vi "Actor Core.vi"(8 "error in":errorcluster, 11 "Square in":refnum<class "Rigol DG822 Square.lvclass">) -> (0 "error out":errorcluster, 3 "Actor out":refnum<class "Actor.lvclass">)   [LabVIEW 2021, in "Rigol DG822 UI.lvlib" / "Rigol DG822 Square.lvlib" / "Rigol DG822 Square.lvclass"]
uses:
  Rigol DG822 Square.lvclass
  D:/LabVIEW/General/Files/lvlibp/Actors.lvlibp/Actors/Actors/Actors.lvclass
  General/Files/lvlibp/Actor Framework.lvlibp/1abvi3w/vi.lib/ActorFramework/Actor/Actor.lvclass
  Rigol DG822 UI/lib/controls.llb/FreqUnitHandler.ctl
  Rigol DG822 UI/lib/controls.llb/DataCluster.ctl
  Rigol DG822 UI/lib/controls.llb/PeriodUnitHandler.ctl
  Rigol DG822 UI/lib/controls.llb/AmplUnitHandler.ctl
  Rigol DG822 UI/lib/controls.llb/HighLUnitHandler.ctl
  Rigol DG822 UI/lib/controls.llb/OffsetUnitHandler.ctl
  Rigol DG822 UI/lib/controls.llb/LowLUnitHandler.ctl
  Rigol DG822 UI/lib/controls.llb/FreqUnit.ctl
  Rigol DG822 UI/lib/controls.llb/PeriodUnit.ctl
  Rigol DG822 UI/lib/controls.llb/AmplUnit.ctl
  Rigol DG822 UI/lib/controls.llb/HighLUnit.ctl
  Rigol DG822 UI/lib/controls.llb/OffsetUnit.ctl
  Rigol DG822 UI/lib/controls.llb/LowLUnit.ctl
  Rigol DG822 UI/lib/controls.llb/WaveformParamTags.ctl
  Rigol DG822 UI/lib/controls.llb/SquareParamDisplay.ctl
  Rigol DG822 UI/lib/controls.llb/SliderControl.ctl
  Rigol DG822 UI/lib/controls.llb/PhaseUnitHandler.ctl
  Rigol DG822 UI/lib/controls.llb/DutyUnitHandler.ctl
  Rigol DG822 UI/lib/controls.llb/StringIndicatorSelected.ctl
  Rigol DG822 UI/lib/controls.llb/RDG822ExtCall.ctl
  Rigol DG822 UI/lib/controls.llb/FT Controls Cluster.ctl
  Rigol DG822 Square.lvclass/Rigol DG822 Square.ctl
  Rigol DG822 UI/lib/controls.llb/WaveformExtCall.ctl
  Rigol DG822 UI/lib/controls.llb/AllWaveformDataCluster.ctl
  Rigol DG822 UI/lib/controls.llb/String Indicators Cluster.ctl
  <vilib>/Utility/miscctls.llb/LVPointTypeDef.ctl
  <userlib>/_MGI/Application Control/MGI VI Reference/MGI Current VI's Reference.vi
  General/Files/lvlibp/Actors.lvlibp/Actors/Actors/Actors.lvclass
panel:
  in  "Slider":T1
  in  "ParamTags":T2
  out "Data":T3={"Freq"={"Freq"=1.0, "FreqUnit"=enum."kHz", "FreqUnitPrcs"=9.0}, "Period"={"Period"=1.0, "PeriodUnit"=enum."ms", "PeriodUnitPrcs"=7.0}, "Ampl"={"Ampl"=5.0, "AmplUnit"=enum."Vpp", "AmplUnitPrcs"=4.0}, "HighL"={"HighL"=2.5, "HighLUnit"=enum."V", "HighLUnitPrcs"=4.0}, "Offset"={"Offset"=0.0, "OffsetUnit"=enum."Vdc", "OffsetUnitPrcs"=4.0}, "LowL"={"LowL"=-2.5, "LowLUnit"=enum."V", "LowLUnitPrcs"=4.0}, "Phase"={"Phase"=0.0, "PhaseUnit"=enum."°", "PhaseUnitPrcs"=3.0}, "Duty"={"Duty"=50.0, "DutyUnit"=enum."%", "DutyUnitPrcs"=3.0}, "Width"={"Width"=500.0, "WidthUnit"=enum."us", "WidthUnitPrcs"=4.0}, "RisEdge"={"RisEdge"=10.0, "RisEdgeUnit"=enum."ns", "RisEdgeUnitPrcs"=1.0}, "FallEdge"={"FallEdge"=10.0, "FallEdgeUnit"=enum."ns", "FallEdgeUnitPrcs"=1.0}} {"RisEdge"."RisEdge" format="%.1f"; "RisEdge"."RisEdgeUnitPrcs" format="%#_1g"; "FallEdge"."FallEdge" format="%.1f"; "FallEdge"."FallEdgeUnitPrcs" format="%#_1g"; "Width"."Width" format="%.4g"; "Width"."WidthUnitPrcs" format="%#_1g"; "Duty"."Duty" format="%.3g"; "Duty"."DutyUnitPrcs" format="%#_1g"; "Phase"."Phase" format="%.3g"; "Phase"."PhaseUnitPrcs" format="%#_1g"; "LowL"."LowL" format="%.4g"; "LowL"."LowLUnitPrcs" format="%#_1g"; "Offset"."Offset" format="%.4g"; "Offset"."OffsetUnitPrcs" format="%#_1g"; "HighL"."HighL" format="%.4g"; "HighL"."HighLUnitPrcs" format="%#_1g"; "Ampl"."Ampl" format="%.4g"; "Ampl"."AmplUnitPrcs" format="%#_1g"; "Period"."Period" format="%.7g"; "Period"."PeriodUnitPrcs" format="%#_1g"; "Freq"."FreqUnitPrcs" format="%#_1g"; "Freq"."Freq" format="%.9g"}
  in  "Conf Tabs":enum32{"Square", "OK"}(tab)
  in  "Slider Tab":enum32{"First", "Second"}(tab)
  in  "F/T Ctrls":T4
  out "String Indcs":T5={"Freq-Period"="1.000,000,000 kHz", "Ampl-HighL"="5.000,0 Vpp", "Offset-LowL"="0.000,0 Vdc", "Phase"="0.000 °"}
  out "F/T Ctrls 2":cluster{"Pict Ring":u16}
  out "String Indcs 2":cluster{"Duty":string}={"Duty"="50.000 %"}
  out "SquareParamDisplay":T6
  in  "Value":dbl=1.0 format="%.8g"
  in  "Unit Tabs":T7(tab)
  out "FreqUnitHandler":T8=1
  in  "FreqUnit":T9=enum."kHz"
  out "PeriodUnitHandler":T10=1
  in  "PeriodUnit":T11=enum."ms"
  in  "AmplUnit":T12=enum."Vpp"
  out "AmplUnitHandler":T13
  out "HighLUnitHandler":T14
  in  "HighLUnit":T15=enum."V"
  out "OffsetUnitHandler":T16
  in  "OffsetUnit":T17=enum."Vdc"
  out "LowLUnitHandler":T18
  in  "LowLUnit":T19=enum."V"
  out "PhaseUnitHandler":T20
  out "DutyUnitHandler":T21
  in  "OK":bool
  # "MHz - 10 \nkHz - 9\nHz - 6\nmHz - 3\nuHz - 0?"
  # "s - 10\nms - 7\nus - 4 \nns - 1?"
  # "All 4 - V - 4\n        mV - 1"
  # "no change"
  # "no change"
  # "s - 10\nms - 7\nus - 4 \nns - 1?"
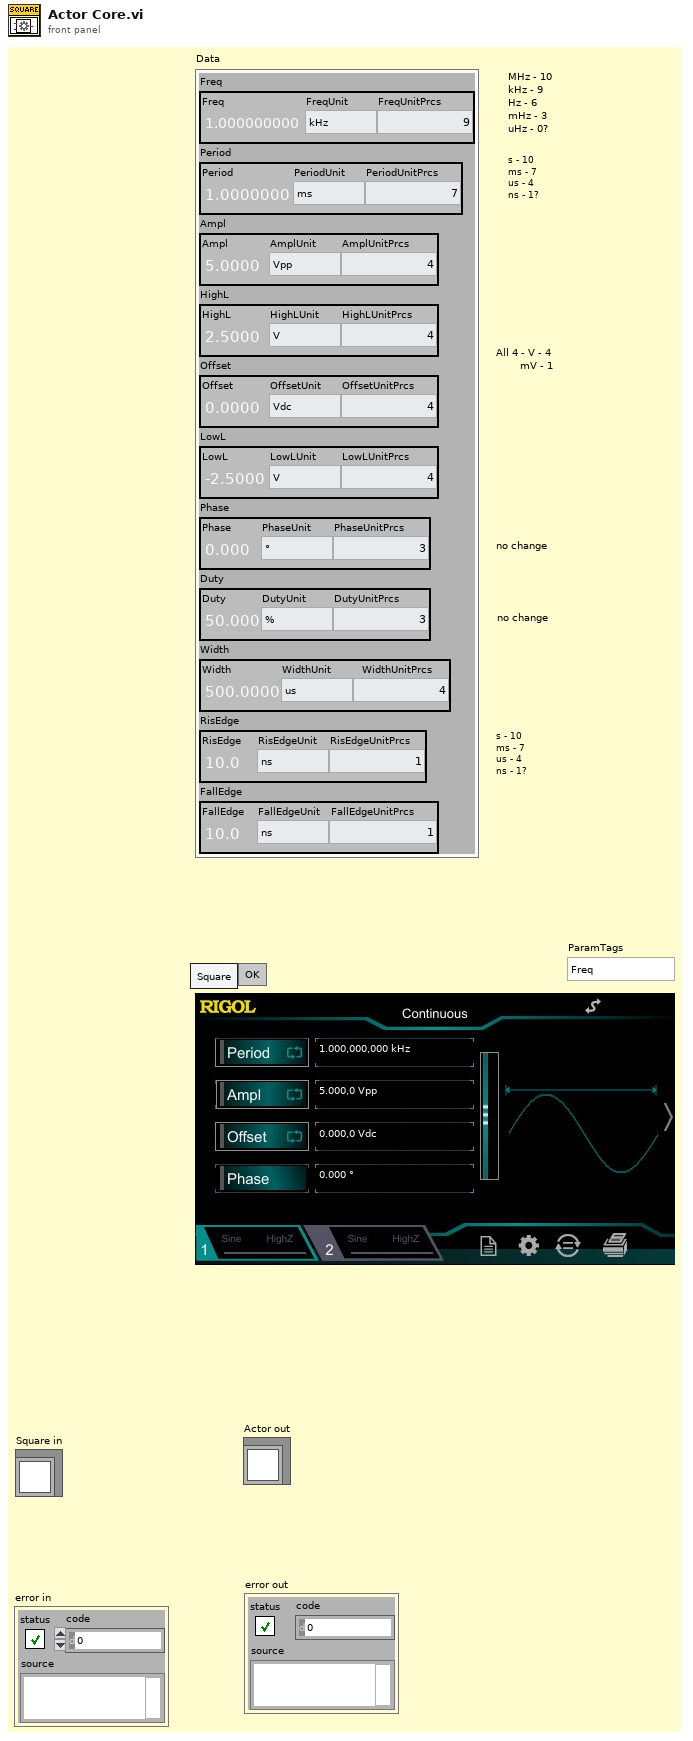
[diagram p1: front panel]
types:
  T1 = typedef "SliderControl.ctl" = bool
  T2 = typedef "WaveformParamTags.ctl" = enum16{"Freq", "Period", "Ampl", "HighL", "Offset", "LowL", "Phase", "Duty", "Width", "RisEdge", "FallEdge"}
  T3 = typedef "DataCluster.ctl" = cluster{"Freq":cluster{"Freq":dbl, "FreqUnit":enum32{"No Selection", "MHz", "kHz", "Hz", "mHz", "uHz"}, "FreqUnitPrcs":dbl}, "Period":cluster{"Period":dbl, "PeriodUnit":enum32{"No Selection", "s", "ms", "us", "ns"}, "PeriodUnitPrcs":dbl}, "Ampl":cluster{"Ampl":dbl, "AmplUnit":enum32{"No Selection", "Vpp", "mVpp"}, "AmplUnitPrcs":dbl}, "HighL":cluster{"HighL":dbl, "HighLUnit":enum32{"No Selection", "V", "mV"}, "HighLUnitPrcs":dbl}, "Offset":cluster{"Offset":dbl, "OffsetUnit":enum32{"No Selection", "Vdc", "mVdc"}, "OffsetUnitPrcs":dbl}, "LowL":cluster{"LowL":dbl, "LowLUnit":enum32{"No Selection", "V", "mV"}, "LowLUnitPrcs":dbl}, "Phase":cluster{"Phase":dbl, "PhaseUnit":enum32{"°"}, "PhaseUnitPrcs":dbl}, "Duty":cluster{"Duty":dbl, "DutyUnit":enum32{"%"}, "DutyUnitPrcs":dbl}, "Width":cluster{"Width":dbl, "WidthUnit":enum32{"No Selection", "s", "ms", "us", "ns"}, "WidthUnitPrcs":dbl}, "RisEdge":cluster{"RisEdge":dbl, "RisEdgeUnit":enum32{"No Selection", "s", "ms", "us", "ns"}, "RisEdgeUnitPrcs":dbl}, "FallEdge":cluster{"FallEdge":dbl, "FallEdgeUnit":enum32{"No Selection", "s", "ms", "us", "ns"}, "FallEdgeUnitPrcs":dbl}}
  T4 = cluster{"Freq/Period":bool, "Ampl/HighL":bool, "Offset/LowL":bool}
  T5 = cluster{"Freq-Period":string, "Ampl-HighL":string, "Offset-LowL":string, "Phase":string}
  T6 = typedef "SquareParamDisplay.ctl" = u16
  T7 = enum32{"Freq", "Period", "Ampl", "HighL", "Offset", "LowL", "Phase", "Duty"}
  T8 = typedef "FreqUnitHandler.ctl" = u16
  T9 = typedef "FreqUnit.ctl" = enum32{"No Selection", "MHz", "kHz", "Hz", "mHz", "uHz"}
  T10 = typedef "PeriodUnitHandler.ctl" = u16
  T11 = typedef "PeriodUnit.ctl" = enum32{"No Selection", "s", "ms", "us", "ns"}
  T12 = typedef "AmplUnit.ctl" = enum32{"No Selection", "Vpp", "mVpp"}
  T13 = typedef "AmplUnitHandler.ctl" = u16
  T14 = typedef "HighLUnitHandler.ctl" = u16
  T15 = typedef "HighLUnit.ctl" = enum32{"No Selection", "V", "mV"}
  T16 = typedef "OffsetUnitHandler.ctl" = u16
  T17 = typedef "OffsetUnit.ctl" = enum32{"No Selection", "Vdc", "mVdc"}
  T18 = typedef "LowLUnitHandler.ctl" = u16
  T19 = typedef "LowLUnit.ctl" = enum32{"No Selection", "V", "mV"}
  T20 = typedef "PhaseUnitHandler.ctl" = u16
  T21 = typedef "DutyUnitHandler.ctl" = u16
  T22 = cluster{"Freq-Period":string, "Freq-Period 2":string, "Freq-Period 3":string, "Freq-Period 4":string, "Freq-Period 5":string}
  T23 = typedef "LVPointTypeDef.ctl" = cluster{"Horizontal":i16, "Vertical":i16}
  T24 = typedef "StringIndicatorSelected.ctl" = enum16{"Freq-Period", "Ampl-HighL", "Offset-LowL", "Phase", "Duty-Width", "RisEdge", "FallEdge"}
  T25 = typedef "FT Controls Cluster.ctl" = cluster{"Freq/Period":bool, "Ampl/HighL":bool, "Offset/LowL":bool, "Duty/Width":bool}
  T26 = typedef "RDG822ExtCall.ctl" = enum16{"Get Data"}
  T27 = typedef "WaveformExtCall.ctl" = enum16{"Freq", "Period", "Ampl", "HighL", "Offset", "LowL", "Phase", "Duty", "Width", "RisEdge", "FallEdge", "Home", "InitData"}
  T28 = cluster{"Freq":cluster{"Freq":dbl, "FreqUnit":enum32{"No Selection", "MHz", "kHz", "Hz", "mHz", "uHz"}, "FreqUnitPrcs":dbl}, "Period":cluster{"Period":dbl, "PeriodUnit":enum32{"No Selection", "s", "ms", "us", "ns"}, "PeriodUnitPrcs":dbl}, "Duty":cluster{"Duty":dbl, "DutyUnit":enum32{"%"}, "DutyUnitPrcs":dbl}}
  T29 = cluster{"Ampl":cluster{"Ampl":dbl, "AmplUnit":enum32{"No Selection", "Vpp", "mVpp"}, "AmplUnitPrcs":dbl}, "HighL":cluster{"HighL":dbl, "HighLUnit":enum32{"No Selection", "V", "mV"}, "HighLUnitPrcs":dbl}, "Offset":cluster{"Offset":dbl, "OffsetUnit":enum32{"No Selection", "Vdc", "mVdc"}, "OffsetUnitPrcs":dbl}, "LowL":cluster{"LowL":dbl, "LowLUnit":enum32{"No Selection", "V", "mV"}, "LowLUnitPrcs":dbl}}
  T30 = cluster{"Phase":dbl, "PhaseUnit":enum32{"°"}, "PhaseUnitPrcs":dbl}
  T31 = cluster{"Duty":dbl, "DutyUnit":enum32{"%"}, "DutyUnitPrcs":dbl}
  T32 = typedef "AllWaveformDataCluster.ctl" = cluster{"Data":T3, "F/T Ctrls":T25, "String Indcs":T33}
  T33 = typedef "String Indicators Cluster.ctl" = cluster{"Freq-Period":string, "Ampl-HighL":string, "Offset-LowL":string, "Phase":string, "Duty-Width":string, "RisEdge":string, "FallEdge":string}
  T34 = enum32{"No Selection", "MHz", "kHz", "Hz", "mHz", "uHz"}
  T35 = cluster{"Value":dbl, "PeriodUnit":u32, "FreqUnitPrecision":dbl}
  T36 = cluster{"Freq":dbl, "FreqUnit":enum32{"No Selection", "MHz", "kHz", "Hz", "mHz", "uHz"}, "FreqUnitPrcs":dbl}
  T37 = cluster{"Period":dbl, "PeriodUnit":enum32{"No Selection", "s", "ms", "us", "ns"}, "PeriodUnitPrcs":dbl}
  T38 = cluster{"Ampl":dbl, "AmplUnit":enum32{"No Selection", "Vpp", "mVpp"}, "AmplUnitPrcs":dbl}
  T39 = cluster{"HighL":dbl, "HighLUnit":enum32{"No Selection", "V", "mV"}, "HighLUnitPrcs":dbl}
  T40 = cluster{"Offset":dbl, "OffsetUnit":enum32{"No Selection", "Vdc", "mVdc"}, "OffsetUnitPrcs":dbl}
  T41 = cluster{"LowL":dbl, "LowLUnit":enum32{"No Selection", "V", "mV"}, "LowLUnitPrcs":dbl}
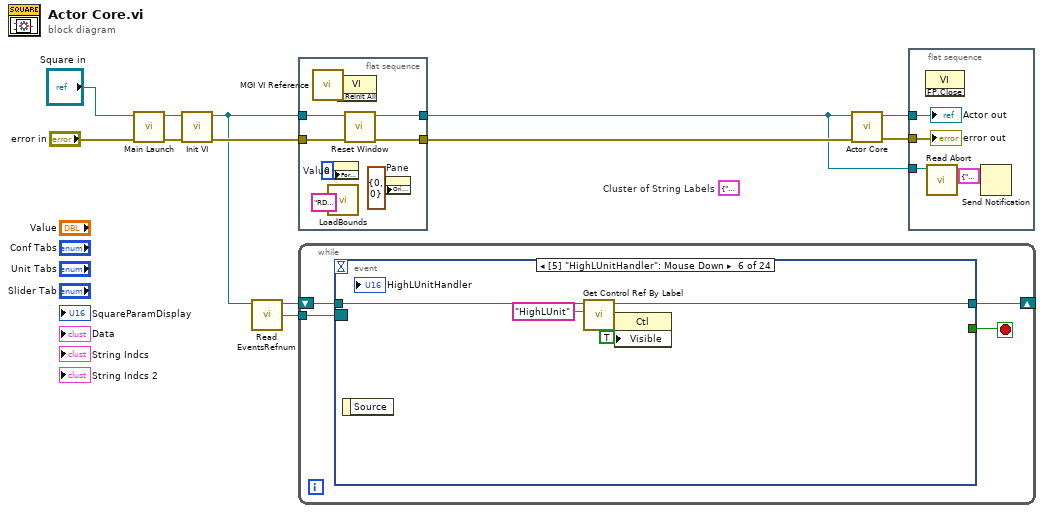
[diagram p0: block diagram]
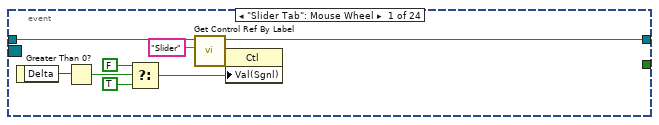
[diagram p2: hidden frame]
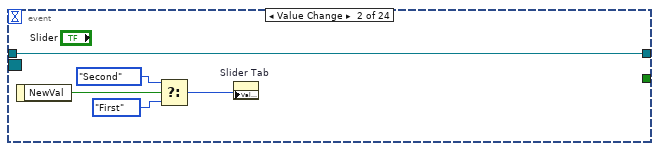
[diagram p3: hidden frame]
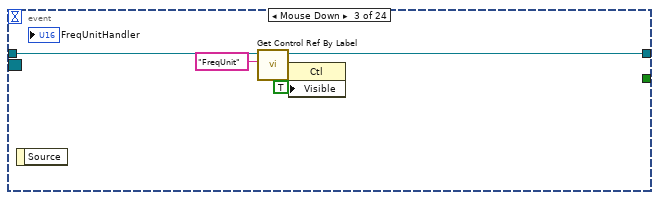
[diagram p4: hidden frame]
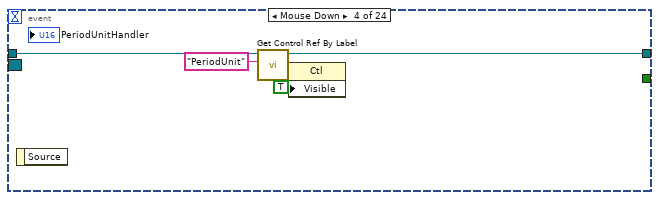
[diagram p5: hidden frame]
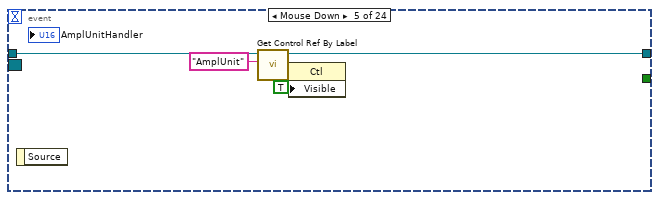
[diagram p6: hidden frame]
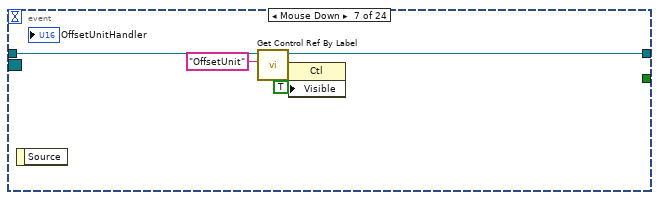
[diagram p7: hidden frame]
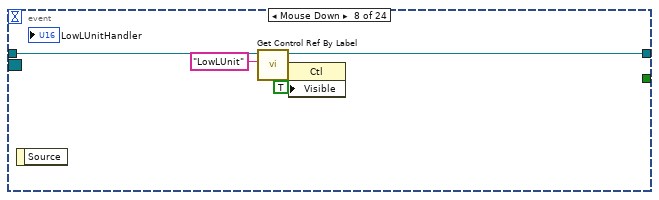
[diagram p8: hidden frame]
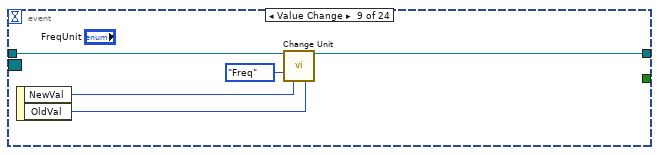
[diagram p9: hidden frame]
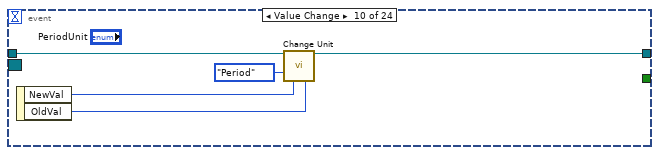
[diagram p10: hidden frame]
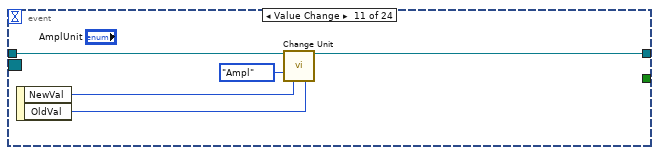
[diagram p11: hidden frame]
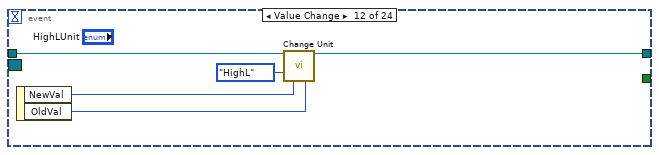
[diagram p12: hidden frame]
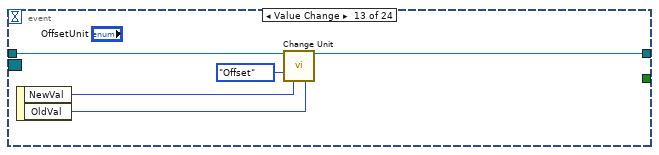
[diagram p13: hidden frame]
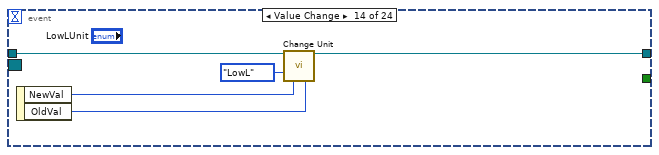
[diagram p14: hidden frame]
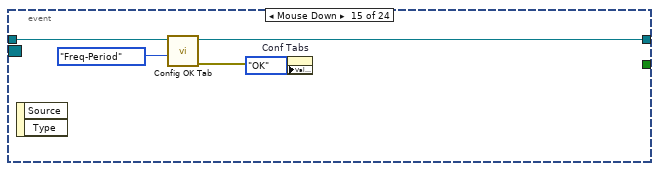
[diagram p15: hidden frame]
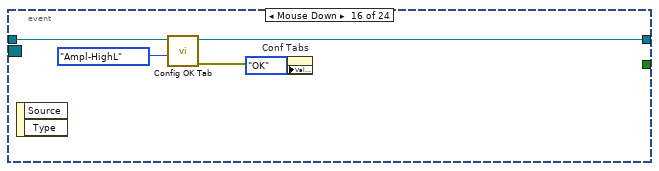
[diagram p16: hidden frame]
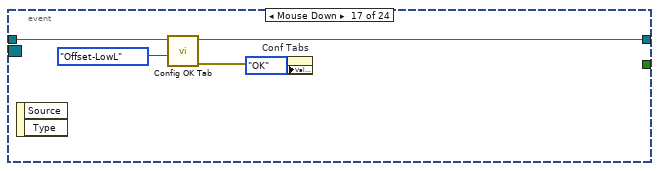
[diagram p17: hidden frame]
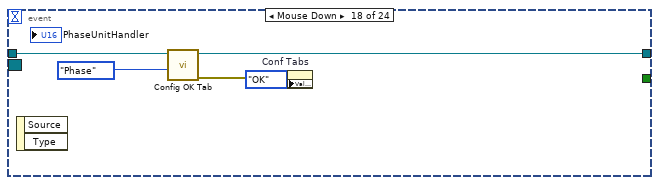
[diagram p18: hidden frame]
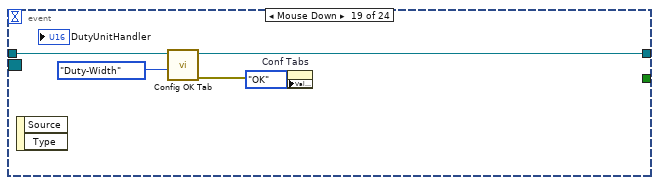
[diagram p19: hidden frame]
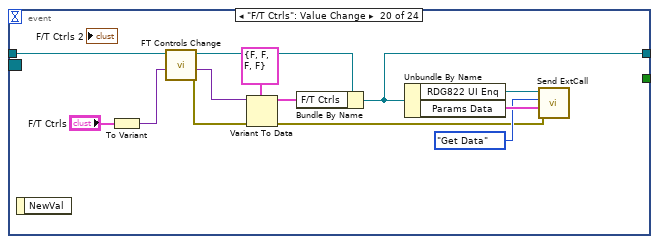
[diagram p20: hidden frame]
diagram:
  (unwired) T22 {"Freq-Period"="String Indcs.Freq-Period", "Freq-Period 2"="String Indcs.Ampl-HighL", "Freq-Period 3"="String Indcs.Offset-LowL", "Freq-Period 4"="String Indcs.Phase", "Freq-Period 5"="String Indcs 2.Duty"}  # Cluster of String Labels
  n1 = call "Main Launch.vi"("error in (no error)"="error in", "Actors in"="Square in") -> ("error out"=w4:errorcluster, "Actors out"=w3:refnum<class "Rigol DG822 Square.lvclass">)  [unwired: 6 in, 2 out]
  n2 = call-dynamic "Init VI.vi"("error in (no error)"=w4, "Rigol DG822 Square in"=w3) -> ("error out"=w5:errorcluster, "Rigol DG822 Square out"=w2:refnum<class "Rigol DG822 Square.lvclass">)  [unwired: 8 in]
  n3 = call "Read EventsRefnum.vi"("Actors in"=w2) -> ("EventsRefnum"=w8:refnum<event-registration>, "Actors out"=w7:refnum<class "Rigol DG822 Square.lvclass">)  [unwired: 9 in]
  n4 = flat-sequence {
    tunnel: w5 -> [w15]
    tunnel: [w18] -> w10
    tunnel: w2 -> [w16]
    tunnel: [w17] -> w6
    frame #0 {
      n5 = call-poly <userlib>:"MGI VI Reference.vi"() -> ("Current VI's Reference"=w14:refnum<vi>)  [unwired: 1 in]
      n6 = call "LoadBounds.vi"("SettingName"="RDG822Square.bounds") -> ()
      n7 = property on="Value" class="DigNum (strict)"("Format"=u8 0 ("Display Format:Format")) -> ()  [unwired: 2 in, 2 out]
      n8 = invoke class="VI" method="Default Vals.Reinit All"(reference=w14) -> ()  [unwired: 2 in, 3 out]
      n9 = call-dynamic "Reset Window.vi"("error in (no error)"=w15, "Rigol DG822 Square in"=w16) -> ("error out"=w18:errorcluster, "Rigol DG822 Square out"=w17:refnum<class "Rigol DG822 Square.lvclass">)  [unwired: 8 in]
      n10 = property on="Pane" class="Pane"("Origin"=T23 {"Horizontal"=0, "Vertical"=0}) -> ()  [unwired: 2 in, 2 out]
    }
  }
  n11 = while {
    tunnel: w8 -> [w24]
    shift-right: [w22] -> _
    shift-left: w7 -> [w23]
    stop <- w21 stop-if-true
    n12 = event shown="[5] \"HighLUnitHandler\": Mouse Down" {
      selector: w24 -> [_ _ _ _ _ _ _ _ _ _ _ _ _ _ _ _ _ _ _ _ _ _ _ w274]
      dyn-events: _ -> [_ _ _ _ _ _ _ _ _ _ _ _ _ _ _ _ _ _ _ _ _ _ _ _]
      timeout: _ -> [_ _ _ _ _ _ _ _ _ _ _ _ _ _ _ _ _ _ _ _ _ _ _ _]
      tunnel: w23 -> [w25 w39 w45 w51 w57 w63 w69 w75 w80 w85 w90 w95 w100 w105 w106 w114 w119 w124 w129 w134 w154 w189 w262 w272]
      tunnel: [w26 w39 w44 w50 w56 w62 w68 w74 w79 w84 w89 w94 w99 w104 w110 w115 w120 w125 w130 w135 w148 w190 w259 w270] -> w22
      tunnel: [_ _ _ _ _ _ _ _ _ _ _ _ _ _ _ _ _ _ _ _ _ _ _ w275] -> w21
      event "Slider Tab": Mouse Wheel {
        n13 = event-data() -> ("Delta"=w34:i32)  [unwired: 1 in]
        n14 = Greater Than 0?(x=w34) -> (x > 0?=w33:bool)
        n15 = Select(t=FALSE, s=w33, f=TRUE) -> (s? t:f=w27:bool)
        n16 = call "Get Control Ref By Label.vi"("Control Label"="Slider", "Actors in"=w25) -> ("error out"=w29:errorcluster, "Control Ref"=w30:refnum<vi>, "Actors out"=w26:refnum<class "Rigol DG822 Square.lvclass">)  [unwired: 7 in]
        n17 = property class="Ctl"(reference=w30, error in=w29, "Val(Sgnl)"=w27) -> ()  [unwired: 2 out]
      }
      event Value Change {
        n18 = event-data() -> ("NewVal"=w35:T1)  [unwired: 1 in]
        n19 = Select(t=enum32{"First", "Second"}."Second" ("Slider Tab"), s=w35, f=enum32{"First", "Second"}."First" ("Slider Tab")) -> (s? t:f=w36:enum32{"First", "Second"})
        n20 = property on="Slider Tab" class="TabCtl (strict)"("Value"=w36) -> ()  [unwired: 2 in, 2 out]
      }
      event Mouse Down {
        n21 = event-data() -> ()  [unwired: 1 in, 1 out]
        n22 = call "Get Control Ref By Label.vi"("Control Label"="FreqUnit", "Actors in"=w45) -> ("error out"=w40:errorcluster, "Control Ref"=w42:refnum<vi>, "Actors out"=w44:refnum<class "Rigol DG822 Square.lvclass">)  [unwired: 7 in]
        n23 = property class="Ctl"(reference=w42, error in=w40, "Visible"=TRUE) -> ()  [unwired: 2 out]
      }
      event Mouse Down {
        n24 = event-data() -> ()  [unwired: 1 in, 1 out]
        n25 = call "Get Control Ref By Label.vi"("Control Label"="PeriodUnit", "Actors in"=w51) -> ("error out"=w46:errorcluster, "Control Ref"=w48:refnum<vi>, "Actors out"=w50:refnum<class "Rigol DG822 Square.lvclass">)  [unwired: 7 in]
        n26 = property class="Ctl"(reference=w48, error in=w46, "Visible"=TRUE) -> ()  [unwired: 2 out]
      }
      event Mouse Down {
        n27 = event-data() -> ()  [unwired: 1 in, 1 out]
        n28 = call "Get Control Ref By Label.vi"("Control Label"="AmplUnit", "Actors in"=w57) -> ("error out"=w52:errorcluster, "Control Ref"=w54:refnum<vi>, "Actors out"=w56:refnum<class "Rigol DG822 Square.lvclass">)  [unwired: 7 in]
        n29 = property class="Ctl"(reference=w54, error in=w52, "Visible"=TRUE) -> ()  [unwired: 2 out]
      }
      event Mouse Down {
        n30 = event-data() -> ()  [unwired: 1 in, 1 out]
        n31 = call "Get Control Ref By Label.vi"("Control Label"="HighLUnit", "Actors in"=w63) -> ("error out"=w58:errorcluster, "Control Ref"=w60:refnum<vi>, "Actors out"=w62:refnum<class "Rigol DG822 Square.lvclass">)  [unwired: 7 in]
        n32 = property class="Ctl"(reference=w60, error in=w58, "Visible"=TRUE) -> ()  [unwired: 2 out]
      }
      event Mouse Down {
        n33 = event-data() -> ()  [unwired: 1 in, 1 out]
        n34 = call "Get Control Ref By Label.vi"("Control Label"="OffsetUnit", "Actors in"=w69) -> ("error out"=w64:errorcluster, "Control Ref"=w66:refnum<vi>, "Actors out"=w68:refnum<class "Rigol DG822 Square.lvclass">)  [unwired: 7 in]
        n35 = property class="Ctl"(reference=w66, error in=w64, "Visible"=TRUE) -> ()  [unwired: 2 out]
      }
      event Mouse Down {
        n36 = event-data() -> ()  [unwired: 1 in, 1 out]
        n37 = call "Get Control Ref By Label.vi"("Control Label"="LowLUnit", "Actors in"=w75) -> ("error out"=w70:errorcluster, "Control Ref"=w72:refnum<vi>, "Actors out"=w74:refnum<class "Rigol DG822 Square.lvclass">)  [unwired: 7 in]
        n38 = property class="Ctl"(reference=w72, error in=w70, "Visible"=TRUE) -> ()  [unwired: 2 out]
      }
      event Value Change {
        n39 = event-data() -> ("NewVal"=w78:T9, "OldVal"=w77:T9)  [unwired: 1 in]
        n40 = call-dynamic "Change Unit.vi"("Rigol DG822 Square in"=w80, "ParamTags"=WaveformParamTags."Freq", "New Value"=w78, "Old Value"=w77) -> ("Rigol DG822 Square out"=w79:refnum<class "Rigol DG822 Square.lvclass">)  [unwired: 10 in, 1 out]
      }
      event Value Change {
        n41 = event-data() -> ("NewVal"=w83:T11, "OldVal"=w82:T11)  [unwired: 1 in]
        n42 = call-dynamic "Change Unit.vi"("Rigol DG822 Square in"=w85, "ParamTags"=WaveformParamTags."Period", "New Value"=w83, "Old Value"=w82) -> ("Rigol DG822 Square out"=w84:refnum<class "Rigol DG822 Square.lvclass">)  [unwired: 10 in, 1 out]
      }
      event Value Change {
        n43 = event-data() -> ("NewVal"=w88:T12, "OldVal"=w87:T12)  [unwired: 1 in]
        n44 = call-dynamic "Change Unit.vi"("Rigol DG822 Square in"=w90, "ParamTags"=WaveformParamTags."Ampl", "New Value"=w88, "Old Value"=w87) -> ("Rigol DG822 Square out"=w89:refnum<class "Rigol DG822 Square.lvclass">)  [unwired: 10 in, 1 out]
      }
      event Value Change {
        n45 = event-data() -> ("NewVal"=w93:T15, "OldVal"=w92:T15)  [unwired: 1 in]
        n46 = call-dynamic "Change Unit.vi"("Rigol DG822 Square in"=w95, "ParamTags"=WaveformParamTags."HighL", "New Value"=w93, "Old Value"=w92) -> ("Rigol DG822 Square out"=w94:refnum<class "Rigol DG822 Square.lvclass">)  [unwired: 10 in, 1 out]
      }
      event Value Change {
        n47 = event-data() -> ("NewVal"=w98:T17, "OldVal"=w97:T17)  [unwired: 1 in]
        n48 = call-dynamic "Change Unit.vi"("Rigol DG822 Square in"=w100, "ParamTags"=WaveformParamTags."Offset", "New Value"=w98, "Old Value"=w97) -> ("Rigol DG822 Square out"=w99:refnum<class "Rigol DG822 Square.lvclass">)  [unwired: 10 in, 1 out]
      }
      event Value Change {
        n49 = event-data() -> ("NewVal"=w103:T19, "OldVal"=w102:T19)  [unwired: 1 in]
        n50 = call-dynamic "Change Unit.vi"("Rigol DG822 Square in"=w105, "ParamTags"=WaveformParamTags."LowL", "New Value"=w103, "Old Value"=w102) -> ("Rigol DG822 Square out"=w104:refnum<class "Rigol DG822 Square.lvclass">)  [unwired: 10 in, 1 out]
      }
      event "String Indcs.Freq-Period": Mouse Down {
        n51 = event-data() -> ()  [unwired: 1 in, 2 out]
        n52 = call-dynamic "Config OK Tab.vi"("String Selected"=StringIndicatorSelected."Freq-Period", "Rigol DG822 Square in"=w106) -> ("error out"=w109:errorcluster, "Rigol DG822 Square out"=w110:refnum<class "Rigol DG822 Square.lvclass">)  [unwired: 8 in]
        n53 = property on="Conf Tabs" class="TabCtl (strict)"(error in=w109, "Value"=enum32{"Square", "OK"}."OK" ("Conf Tabs")) -> ()  [unwired: 1 in, 2 out]
      }
      event "String Indcs.Ampl-HighL": Mouse Down {
        n54 = event-data() -> ()  [unwired: 1 in, 2 out]
        n55 = call-dynamic "Config OK Tab.vi"("String Selected"=StringIndicatorSelected."Ampl-HighL", "Rigol DG822 Square in"=w114) -> ("error out"=w113:errorcluster, "Rigol DG822 Square out"=w115:refnum<class "Rigol DG822 Square.lvclass">)  [unwired: 8 in]
        n56 = property on="Conf Tabs" class="TabCtl (strict)"(error in=w113, "Value"=enum32{"Square", "OK"}."OK" ("Conf Tabs")) -> ()  [unwired: 1 in, 2 out]
      }
      event "String Indcs.Offset-LowL": Mouse Down {
        n57 = event-data() -> ()  [unwired: 1 in, 2 out]
        n58 = call-dynamic "Config OK Tab.vi"("String Selected"=StringIndicatorSelected."Offset-LowL", "Rigol DG822 Square in"=w119) -> ("error out"=w118:errorcluster, "Rigol DG822 Square out"=w120:refnum<class "Rigol DG822 Square.lvclass">)  [unwired: 8 in]
        n59 = property on="Conf Tabs" class="TabCtl (strict)"(error in=w118, "Value"=enum32{"Square", "OK"}."OK" ("Conf Tabs")) -> ()  [unwired: 1 in, 2 out]
      }
      event "String Indcs.Phase": Mouse Down {
        n60 = event-data() -> ()  [unwired: 1 in, 2 out]
        n61 = call-dynamic "Config OK Tab.vi"("String Selected"=StringIndicatorSelected."Phase", "Rigol DG822 Square in"=w124) -> ("error out"=w123:errorcluster, "Rigol DG822 Square out"=w125:refnum<class "Rigol DG822 Square.lvclass">)  [unwired: 8 in]
        n62 = property on="Conf Tabs" class="TabCtl (strict)"(error in=w123, "Value"=enum32{"Square", "OK"}."OK" ("Conf Tabs")) -> ()  [unwired: 1 in, 2 out]
      }
      event "String Indcs 2.Duty": Mouse Down {
        n63 = event-data() -> ()  [unwired: 1 in, 2 out]
        n64 = call-dynamic "Config OK Tab.vi"("String Selected"=StringIndicatorSelected."Duty-Width", "Rigol DG822 Square in"=w129) -> ("error out"=w128:errorcluster, "Rigol DG822 Square out"=w130:refnum<class "Rigol DG822 Square.lvclass">)  [unwired: 8 in]
        n65 = property on="Conf Tabs" class="TabCtl (strict)"(error in=w128, "Value"=enum32{"Square", "OK"}."OK" ("Conf Tabs")) -> ()  [unwired: 1 in, 2 out]
      }
      event "F/T Ctrls": Value Change {
        n66 = event-data() -> ()  [unwired: 1 in, 1 out]
        n67 = To Variant(anything="F/T Ctrls") -> (Variant=w133:variant)
        n68 = call-dynamic "FT Controls Change.vi"("F/T Controls Cluster Variant"=w133, "Rigol DG822 Square in"=w134) -> ("error out"=w138:errorcluster, "New F/T Controls Cluster Variant"=w142:variant, "Rigol DG822 Square out"=w143:refnum<class "Rigol DG822 Square.lvclass">)  [unwired: 7 in]
        n69 = Variant To Data(error in=w138, type=T25 {"Freq/Period"=FALSE, "Ampl/HighL"=FALSE, "Offset/LowL"=FALSE, "Duty/Width"=FALSE} ("F/T Ctrls"), Variant=w142) -> (data=w141:T25, error out=w132:errorcluster)
        n70 = Bundle By Name(cluster=w143, "F/T Ctrls"=w141) -> (w135:refnum<class "Rigol DG822 Square.lvclass">)
        n71 = Unbundle By Name(w135) -> ("RDG822 UI Enq"=w140:refnum<class "Message Enqueuer.lvclass">, "Params Data"=w139:T32)
        n72 = call "Send ExtCall.vi"("error in (no error)"=w132, "Val"=w139, "Tag"=RDG822ExtCall."Get Data", "Message Enqueuer"=w140) -> ()  [unwired: 4 in, 4 out]
      }
      event "OK": Value Change {
        n73 = event-data() -> ()  [unwired: 1 in, 2 out]
        n74 = case shown="\"Freq\"" "ParamTags" {
          tunnel: [w160 w163 w166 w169 w172 w175 w178 w181 4.0 ("FreqUnitPrecision")] -> w155
          tunnel: [w161 w164 w167 w170 w173 w176 w179 w182 1] -> w156
          tunnel: w154 -> [w159 w162 w165 w168 w171 w174 w177 w180 _]
          frame "Freq" {
            n75 = Unbundle By Name(w159) -> ("FreqUnit"=w161:T34, "FreqUnitPrcs"=w160:dbl)
          }
          frame "Period" {
            n76 = Unbundle By Name(w162) -> ("PeriodUnit"=w164:enum32{"No Selection", "s", "ms", "us", "ns"}, "PeriodUnitPrcs"=w163:dbl)
          }
          frame "Ampl" {
            n77 = Unbundle By Name(w165) -> ("AmplUnit"=w167:enum32{"No Selection", "Vpp", "mVpp"}, "AmplUnitPrcs"=w166:dbl)
          }
          frame "HighL" {
            n78 = Unbundle By Name(w168) -> ("HighLUnit"=w170:enum32{"No Selection", "V", "mV"}, "HighLUnitPrcs"=w169:dbl)
          }
          frame "Offset" {
            n79 = Unbundle By Name(w171) -> ("OffsetUnit"=w173:enum32{"No Selection", "Vdc", "mVdc"}, "OffsetUnitPrcs"=w172:dbl)
          }
          frame "LowL" {
            n80 = Unbundle By Name(w174) -> ("LowLUnit"=w176:enum32{"No Selection", "V", "mV"}, "LowLUnitPrcs"=w175:dbl)
          }
          frame "Phase" {
            n81 = Unbundle By Name(w177) -> ("PhaseUnit"=w179:enum32{"°"}, "PhaseUnitPrcs"=w178:dbl)
          }
          frame "Duty" {
            n82 = Unbundle By Name(w180) -> ("DutyUnit"=w182:enum32{"%"}, "DutyUnitPrcs"=w181:dbl)
          }
          frame Default {
          }
        }
        n83 = call "Get Control Ref By Label.vi"("Control Label"="Value", "Actors in"=w154) -> ("error out"=w151:errorcluster, "Control Ref"=w153:refnum<vi>, "Actors out"=w147:refnum<class "Rigol DG822 Square.lvclass">)  [unwired: 7 in]
        n84 = call "Value Round.vi"("error in (no error)"=w151, "UnitPrecision"=w155, "Value Ref"=w153) -> ("error out"=w150:errorcluster, "Value"=w149:dbl)  [unwired: 7 in]
        n85 = Unbundle By Name(w147) -> ("Self Enq"=w158:refnum<class "Message Enqueuer.lvclass">)
        n86 = Bundle("Value"=w149, "PeriodUnit"=w156, "FreqUnitPrecision"=w155) -> (w157:T35)  [unwired: 1 in]
        n87 = call "Send ExtCall.vi"("error in (no error)"=w150, "Val"=w157, "Tag"="ParamTags", "Message Enqueuer"=w158) -> ("error out"=w145:errorcluster)  [unwired: 4 in, 3 out]
        n88 = call "Set Concrol Value.vi"("error in (no error)"=w145, "Value"="ParamTags", "Control Label"="SquareParamDisplay", "Actors in"=w147) -> ("Actors out"=w148:refnum<class "Rigol DG822 Square.lvclass">)  [unwired: 6 in, 1 out]
      }
      event User Event {
        n89 = event-data() -> ("Type"=w187:u16, "Data"=w188:variant)  [unwired: 1 in]
        n90 = Type Cast(type=WaveformExtCall."Freq" ("Enum"), x=w187) -> (*(type *) &x=w186:T27)
        n91 = case shown="\"Home\", Default" w186 {
          selector: w186 -> [w201 w213 w229 w241 _ _]
          tunnel: [w203 w222 w233 w244 w246 w257] -> w190
          tunnel: w189 -> [w202 w214 w228 w240 w247 w255]
          tunnel: w188 -> [w200 w212 w227 w239 _ w258]
          frame "Freq", "Period" {
            n92 = Variant To Data(type=T28 {"Freq"={"Freq"=1.0, "FreqUnit"=enum."kHz", "FreqUnitPrcs"=9.0}, "Period"={"Period"=1.0, "PeriodUnit"=enum."ms", "PeriodUnitPrcs"=7.0}, "Duty"={"Duty"=50.0, "DutyUnit"=enum."%", "DutyUnitPrcs"=3.0}}, Variant=w200) -> (data=w205:T28)  [unwired: 1 in, 1 out]
            n93 = Unbundle(w205) -> ("Freq"=w206:T36, "Period"=w207:T37, "Duty"=w198:T31)
            n94 = Bundle By Name(cluster=w202, "Freq"=w206, "Period"=w207, "Duty"=w198) -> (w204:refnum<class "Rigol DG822 Square.lvclass">)
            n95 = call-dynamic "Update String Values.vi"("Type"=w201, "Rigol DG822 Square in"=w204) -> ("error out"=w196:errorcluster, "Rigol DG822 Square out"=w197:refnum<class "Rigol DG822 Square.lvclass">)  [unwired: 8 in]
            n96 = call-dynamic "Update String Values.vi"("error in (no error)"=w196, "Type"=u16 7, "Rigol DG822 Square in"=w197) -> ("error out"=w193:errorcluster, "Rigol DG822 Square out"=w194:refnum<class "Rigol DG822 Square.lvclass">)  [unwired: 7 in]
            n97 = call-dynamic "Send Data.vi"("error in (no error)"=w193, "Rigol DG822 Square in"=w194) -> ("error out"=w191:errorcluster, "Rigol DG822 Square out"=w192:refnum<class "Rigol DG822 Square.lvclass">)  [unwired: 8 in]
            n98 = call-dynamic "Reset Window.vi"("error in (no error)"=w191, "Rigol DG822 Square in"=w192) -> ("Rigol DG822 Square out"=w203:refnum<class "Rigol DG822 Square.lvclass">)  [unwired: 8 in, 1 out]
          }
          frame "Ampl".."LowL" {
            n99 = Variant To Data(type=T29 {"Ampl"={"Ampl"=5.0, "AmplUnit"=enum."Vpp", "AmplUnitPrcs"=4.0}, "HighL"={"HighL"=2.5, "HighLUnit"=enum."V", "HighLUnitPrcs"=4.0}, "Offset"={"Offset"=0.0, "OffsetUnit"=enum."Vdc", "OffsetUnitPrcs"=4.0}, "LowL"={"LowL"=-2.5, "LowLUnit"=enum."V", "LowLUnitPrcs"=4.0}}, Variant=w212) -> (data=w216:T29)  [unwired: 1 in, 1 out]
            n100 = Unbundle(w216) -> ("Ampl"=w217:T38, "HighL"=w220:T39, "Offset"=w219:T40, "LowL"=w218:T41)
            n101 = Bundle By Name(cluster=w214, "Ampl"=w217, "HighL"=w220, "Offset"=w219, "LowL"=w218) -> (w221:refnum<class "Rigol DG822 Square.lvclass">)
            n102 = call-dynamic "Update String Values.vi"("Type"=w213, "Rigol DG822 Square in"=w221) -> ("error out"=w209:errorcluster, "Rigol DG822 Square out"=w211:refnum<class "Rigol DG822 Square.lvclass">)  [unwired: 8 in]
            n103 = call-dynamic "Send Data.vi"("error in (no error)"=w209, "Rigol DG822 Square in"=w211) -> ("error out"=w208:errorcluster, "Rigol DG822 Square out"=w210:refnum<class "Rigol DG822 Square.lvclass">)  [unwired: 8 in]
            n104 = call-dynamic "Reset Window.vi"("error in (no error)"=w208, "Rigol DG822 Square in"=w210) -> ("Rigol DG822 Square out"=w222:refnum<class "Rigol DG822 Square.lvclass">)  [unwired: 8 in, 1 out]
          }
          frame "Phase" {
            n105 = Variant To Data(type=T30 {"Phase"=0.0, "PhaseUnit"=enum."°", "PhaseUnitPrcs"=3.0} ("Phase"), Variant=w227) -> (data=w232:T30)  [unwired: 1 in, 1 out]
            n106 = Bundle By Name(cluster=w228, "Phase"=w232) -> (w231:refnum<class "Rigol DG822 Square.lvclass">)
            n107 = call-dynamic "Update String Values.vi"("Type"=w229, "Rigol DG822 Square in"=w231) -> ("error out"=w224:errorcluster, "Rigol DG822 Square out"=w225:refnum<class "Rigol DG822 Square.lvclass">)  [unwired: 8 in]
            n108 = call-dynamic "Send Data.vi"("error in (no error)"=w224, "Rigol DG822 Square in"=w225) -> ("error out"=w223:errorcluster, "Rigol DG822 Square out"=w226:refnum<class "Rigol DG822 Square.lvclass">)  [unwired: 8 in]
            n109 = call-dynamic "Reset Window.vi"("error in (no error)"=w223, "Rigol DG822 Square in"=w226) -> ("Rigol DG822 Square out"=w233:refnum<class "Rigol DG822 Square.lvclass">)  [unwired: 8 in, 1 out]
          }
          frame "Duty" {
            n110 = Variant To Data(type=T31 {"Duty"=50.0, "DutyUnit"=enum."%", "DutyUnitPrcs"=3.0} ("Duty"), Variant=w239) -> (data=w243:T31)  [unwired: 1 in, 1 out]
            n111 = Bundle By Name(cluster=w240, "Duty"=w243) -> (w242:refnum<class "Rigol DG822 Square.lvclass">)
            n112 = call-dynamic "Update String Values.vi"("Type"=w241, "Rigol DG822 Square in"=w242) -> ("error out"=w235:errorcluster, "Rigol DG822 Square out"=w236:refnum<class "Rigol DG822 Square.lvclass">)  [unwired: 8 in]
            n113 = call-dynamic "Send Data.vi"("error in (no error)"=w235, "Rigol DG822 Square in"=w236) -> ("error out"=w234:errorcluster, "Rigol DG822 Square out"=w237:refnum<class "Rigol DG822 Square.lvclass">)  [unwired: 8 in]
            n114 = call-dynamic "Reset Window.vi"("error in (no error)"=w234, "Rigol DG822 Square in"=w237) -> ("Rigol DG822 Square out"=w244:refnum<class "Rigol DG822 Square.lvclass">)  [unwired: 8 in, 1 out]
          }
          frame "Home", Default {
            n115 = property on="Conf Tabs" class="TabCtl (strict)"("Value"=enum32{"Square", "OK"}."Square" ("Conf Tabs")) -> (error out=w245:errorcluster)  [unwired: 2 in, 1 out]
            n116 = call-dynamic "Reset Window.vi"("error in (no error)"=w245, "Rigol DG822 Square in"=w247) -> ("Rigol DG822 Square out"=w246:refnum<class "Rigol DG822 Square.lvclass">)  [unwired: 8 in, 1 out]
          }
          frame "InitData" {
            n117 = Variant To Data(type=T32 {"Data"={"Freq"={"Freq"=1.0, "FreqUnit"=enum."kHz", "FreqUnitPrcs"=9.0}, "Period"={"Period"=1.0, "PeriodUnit"=enum."ms", "PeriodUnitPrcs"=7.0}, "Ampl"={"Ampl"=5.0, "AmplUnit"=enum."Vpp", "AmplUnitPrcs"=4.0}, "HighL"={"HighL"=2.5, "HighLUnit"=enum."V", "HighLUnitPrcs"=4.0}, "Offset"={"Offset"=0.0, "OffsetUnit"=enum."Vdc", "OffsetUnitPrcs"=4.0}, "LowL"={"LowL"=-2.5, "LowLUnit"=enum."V", "LowLUnitPrcs"=4.0}, "Phase"={"Phase"=0.0, "PhaseUnit"=enum."°", "PhaseUnitPrcs"=3.0}, "Duty"={"Duty"=50.0, "DutyUnit"=enum."%", "DutyUnitPrcs"=3.0}, "Width"={"Width"=500.0, "WidthUnit"=enum."us", "WidthUnitPrcs"=4.0}, "RisEdge"={"RisEdge"=10.0, "RisEdgeUnit"=enum."ns", "RisEdgeUnitPrcs"=1.0}, "FallEdge"={"FallEdge"=10.0, "FallEdgeUnit"=enum."ns", "FallEdgeUnitPrcs"=1.0}}, "F/T Ctrls"={"Freq/Period"=FALSE, "Ampl/HighL"=FALSE, "Offset/LowL"=FALSE, "Duty/Width"=FALSE}, "String Indcs"={"Freq-Period"="1.000,000,000 kHz", "Ampl-HighL"="5.000,0 Vpp", "Offset-LowL"="0.000,0 Vdc", "Phase"="0.000 °", "Duty-Width"="50.000 %", "RisEdge"="10.0 ns", "FallEdge"="10.0 ns"}} ("Params Data"), Variant=w258) -> (data=w256:T32, error out=w251:errorcluster)  [unwired: 1 in]
            n118 = Bundle By Name(cluster=w255, "Params Data"=w256) -> (w253:refnum<class "Rigol DG822 Square.lvclass">)
            n119 = call-dynamic "Update String Values.vi"("error in (no error)"=w251, "Type"=u16 7, "Rigol DG822 Square in"=w253) -> ("error out"=w250:errorcluster, "Rigol DG822 Square out"=w252:refnum<class "Rigol DG822 Square.lvclass">)  [unwired: 7 in]
            n120 = call-dynamic "Init Data.vi"("error in (no error)"=w250, "Rigol DG822 Square in"=w252) -> ("Rigol DG822 Square out"=w257:refnum<class "Rigol DG822 Square.lvclass">)  [unwired: 8 in, 1 out]
          }
        }
      }
      event Panel Close? {
        n121 = event-data() -> ()  [unwired: 1 in, 1 out]
        n122 = flat-sequence {
          tunnel: w262 -> [w265]
          tunnel: [w265] -> w261
          tunnel: w261 -> [w267]
          tunnel: [w266] -> w260
          tunnel: [TRUE] -> w263
          tunnel: [w268] -> w259
          tunnel: w260 -> [w268]
          frame #0 {
            n123 = call "SaveBounds.vi"("SettingName"="RDG822Square.bounds") -> ()
          }
          frame #1 {
            n124 = call "SetClose.vi"("Actors in"=w267) -> ("Actors out"=w266:refnum<class "Rigol DG822 Square.lvclass">)  [unwired: 9 in, 1 out]
          }
          frame #2 {
          }
        }
        n125 = event-data("Discard?"=w263) -> ()  [unwired: 1 in, 1 out]
      }
      event User Event {
        n126 = event-data() -> ()  [unwired: 1 in, 1 out]
        n127 = flat-sequence {
          tunnel: w274 -> [w277]
          tunnel: [w276] -> w273
          tunnel: w272 -> [w276]
          tunnel: w273 -> [w278]
          tunnel: [w278] -> w271
          tunnel: [TRUE] -> w275
          tunnel: w271 -> [w279]
          tunnel: [w279] -> w270
          frame #0 {
            n128 = Unregister For Events(event registration refnum=w277) -> ()  [unwired: 1 in, 1 out]
          }
          frame #1 {
          }
          frame #2 {
          }
        }
      }
    }
  }
  n129 = call-parent "Actor Core.vi"("error in"=w10, "Actor in"=w6) -> ("error out"=w9:errorcluster, "Actor out"=w1:refnum<class "Actor.lvclass">)  [unwired: 8 in]
  n130 = flat-sequence {
    tunnel: w1 -> [w285]
    tunnel: w9 -> [w284]
    tunnel: w6 -> [w281]
    frame #0 {
      n131 = invoke class="VI" method="FP.Close"() -> ()  [unwired: 3 in, 3 out]
      n132 = call "Read Abort.vi"("Actors in"=w281) -> ("AbortEvent"=w283:refnum<notifier>)  [unwired: 10 in]
      n133 = Send Notification(notification=cluster{"Caller":string, "AnyValue":variant} {"Caller"="abort", "AnyValue"=variant}, notifier=w283) -> ()  [unwired: 1 in, 2 out]
      "Actor out" <- w285
      "error out" <- w284
    }
  }
